vi "saveAvgSpectrum.vi"(7 "No. Averages":i32, 9 "tau":dbl, 10 "pd ts":cluster{dbl, dbl, dbl}, 11 "mic ts":T1) -> (1 "CRD":string[](array[string]), 2 "PD":string[](array[string]), 3 "Mic":string[](array[string]))   [LabVIEW 2011]
uses:
  <vilib>/Analysis/NI_AALBase.lvlib
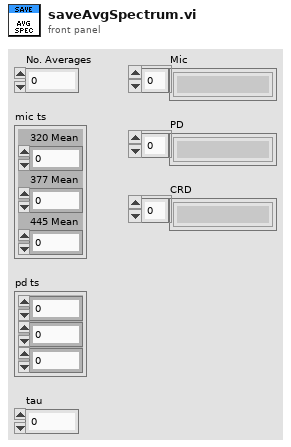
[diagram p1: front panel]
types:
  T1 = cluster{"320 Mean":dbl, "377 Mean":dbl, "445 Mean":dbl}
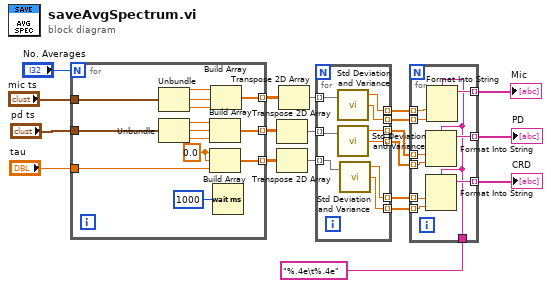
[diagram p0: block diagram]
diagram:
  n1 = for {
    N: "No. Averages" -> [_]
    tunnel: [w32] -> w2 mode=indexing
    tunnel: [w27] -> w6 mode=indexing
    tunnel: [w24] -> w8 mode=indexing
    tunnel: "mic ts" -> [w23]
    tunnel: "pd ts" -> [w22]
    tunnel: "tau" -> [w21]
    w25 = 0.0 ("element")
    n2 = Unbundle(w23) -> ("320 Mean"=w33:dbl, "377 Mean"=w34:dbl, "445 Mean"=w30:dbl)
    n3 = Unbundle(w22) -> (w29:dbl, w28:dbl, w26:dbl)
    n4 = Build Array(w29, w28, w26) -> (w27:dbl[])
    n5 = Build Array(w25, w25, w21) -> (w24:dbl[])
    n6 = Build Array(w33, w34, w30) -> (w32:dbl[])
    n7 = Wait (ms)(milliseconds to wait=u32 1000) -> ()  [unwired: 1 out]
  }
  n8 = Transpose 2D Array(2D array=w6) -> (transposed array=w7:dbl[][])
  n9 = Transpose 2D Array(2D array=w8) -> (transposed array=w9:dbl[][])
  n10 = Transpose 2D Array(2D array=w2) -> (transposed array=w3:dbl[][])
  n11 = for {
    tunnel: w3 -> [w43] mode=indexing
    tunnel: [w42] -> w4 mode=indexing
    tunnel: [w41] -> w5 mode=indexing
    tunnel: w7 -> [w40] mode=indexing
    tunnel: w9 -> [w39] mode=indexing
    tunnel: [w38] -> w13 mode=indexing
    tunnel: [w37] -> w12 mode=indexing
    tunnel: [w36] -> w10 mode=indexing
    tunnel: [w35] -> w11 mode=indexing
    n12 = call <vilib>:"Std Deviation and Variance.vi"("X"=w43) -> ("mean"=w42:dbl, "standard deviation"=w41:dbl)  [unwired: 1 in, 1 out]
    n13 = call <vilib>:"Std Deviation and Variance.vi"("X"=w40) -> ("mean"=w36:dbl, "standard deviation"=w35:dbl)  [unwired: 1 in, 1 out]
    n14 = call <vilib>:"Std Deviation and Variance.vi"("X"=w39) -> ("mean"=w38:dbl, "standard deviation"=w37:dbl)  [unwired: 1 in, 1 out]
  }
  n15 = for {
    tunnel: w4 -> [w53] mode=indexing
    tunnel: w5 -> [w52] mode=indexing
    tunnel: [w47] -> w14 mode=indexing
    tunnel: w10 -> [w51] mode=indexing
    tunnel: w11 -> [w50] mode=indexing
    tunnel: w12 -> [w49] mode=indexing
    tunnel: w13 -> [w48] mode=indexing
    tunnel: [w45] -> w16 mode=indexing
    tunnel: [w46] -> w15 mode=indexing
    tunnel: "%.4e\t%.4e" ("format string") -> [w44]
    n16 = Format Into String(format string=w44, w51, w50) -> (resulting string=w46:string)  [unwired: 2 in, 1 out]
    n17 = Format Into String(format string=w44, w48, w49) -> (resulting string=w45:string)  [unwired: 2 in, 1 out]
    n18 = Format Into String(format string=w44, w53, w52) -> (resulting string=w47:string)  [unwired: 2 in, 1 out]
  }
  "CRD" <- w16
  "PD" <- w15
  "Mic" <- w14
